vi "FS Sketch Spline.vi"(8 "Sketch/Body #":i32=1, 9 "Spline Points":dbl[][](array[numeric]), 10 "Sketch Plane":T1, 11 "Feature In":string="FeatureScript 1247;\nimport(path : \"onshape/std/geometry.fs\", version : \"1247.0\");\n\nannotation { \"Feature Type Name\" : \"LabVIEW Feature\" }\nexport const myFeature = defineFeature(function(context is Context, id is Id, definition is map)\n    precondition\n    {\n        // Define the parameters of the feature type\n    }\n    {\n        // Define the function's action\n    });") -> (3 "Feature Out":string="FeatureScript 1247;\nimport(path : \"onshape/std/geometry.fs\", version : \"1247.0\");\n\nannotation { \"Feature Type Name\" : \"LVFeat1\" }\nexport const myFeature = defineFeature(function(context is Context, id is Id, definition is map)\n    precondition\n    {\n        // Define the parameters of the feature type\n    }\n    {\n        // Define the function's action\n\nvar sketch1 = newSketch(context, id + \"sketch1\", {\n                \"sketchPlane\" : qCreatedBy(makeId(\"Top\"), EntityType.FACE)\n        });\n        // Create sketch entities here\n        skRectangle(sketch1, \"rectangle1\", {\n                \"firstCorner\" : vector(0, 0) * inch,\n                \"secondCorner\" : vector(3, 4) * inch\n        });\n        \n        skSolve(sketch1);\n    });")   [LabVIEW 2019]
uses:
  <userlib>/Onshape Feature Funcrions/_SubVI/Sketch Plane.ctl
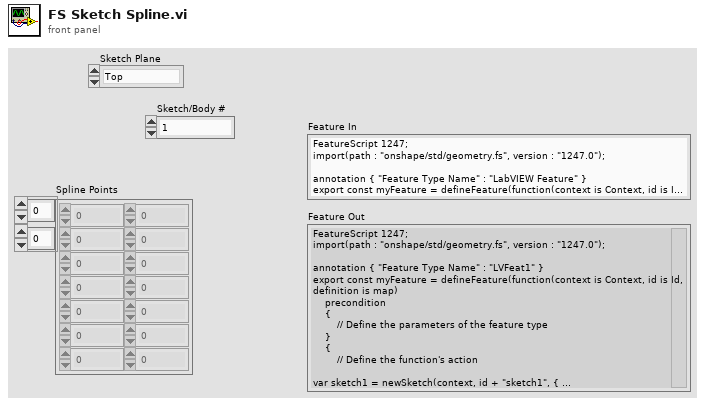
[diagram p1: front panel]
types:
  T1 = typedef "Sketch Plane.ctl" = enum16{"Top", "Front", "Right", "plane1", "plane2", "plane3"}
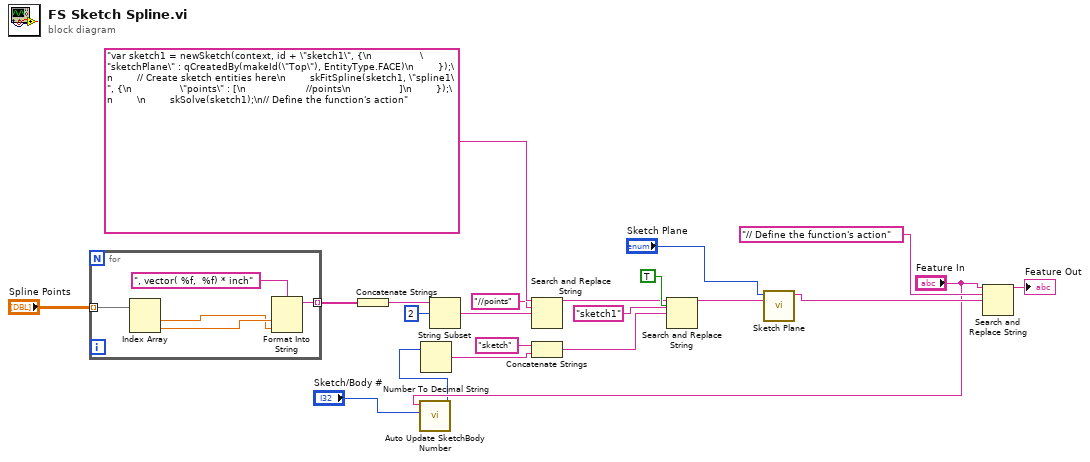
[diagram p0: block diagram]
diagram:
  n1 = for {
    tunnel: "Spline Points" -> [w26] mode=indexing
    tunnel: [w24] -> w10 mode=indexing
    n2 = Index Array(array=w26) -> (element #1=w22:dbl, element #2=w23:dbl)  [unwired: 2 in]
    n3 = Format Into String(format string=", vector( %f,  %f) * inch" ("string"), w23, w22) -> (resulting string=w24:string)  [unwired: 2 in, 1 out]
  }
  n4 = Concatenate Strings(w10) -> (w9:string)
  n5 = call "Auto Update SketchBody Number.vi"("Sketch # in"="Sketch/Body #", "Feature In"="Feature In") -> ("Sketch # out"=w1:i32)  [unwired: 8 in, 1 out]
  n6 = Number To Decimal String(number=w1) -> (decimal integer string=w13:string)  [unwired: 1 in]
  n7 = String Subset(string=w9, offset (0)=2) -> (substring=w7:string)  [unwired: 1 in]
  n8 = Search and Replace String(input string="var sketch1 = newSketch(context, id + \"sketch1\", {\n                \"sketchPlane\" : qCreatedBy(makeId(\"Top\"), EntityType.FACE)\n        });\n        // Create sketch entities here\n        skFitSpline(sketch1, \"spline1\", {\n                \"points\" : [\n                    //points\n                ]\n        });\n        \n        skSolve(sketch1);\n// Define the function's action" ("string"), search string="//points" ("regular expression"), replace string=w7) -> (result string=w11:string)  [unwired: 5 in, 3 out]
  n9 = Concatenate Strings("sketch" ("regular expression"), w13) -> (w14:string)
  n10 = Search and Replace String(replace all?=TRUE ("replace all? (F)"), input string=w11, search string="sketch1" ("regular expression"), replace string=w14) -> (result string=w6:string)  [unwired: 4 in, 3 out]
  n11 = call <userlib>:"Sketch Plane.vi"("result string in"=w6, "Sketch Plane"="Sketch Plane") -> ("result string out"=w4:string)  [unwired: 9 in]
  n12 = Search and Replace String(input string="Feature In", search string="// Define the function's action", replace string=w4) -> (result string=→"Feature Out":string)  [unwired: 5 in, 3 out]
